vi "UniRec.vi"() -> ()   [LabVIEW 2011]
uses:
  <instrlib>/niHWS/nihws.llb/niHWS Open File Permissions ID.ctl
  <vilib>/DAQmx/write.llb/DAQmx Write (Analog Wfm 1Chan NSamp).vi
  <vilib>/DAQmx/read.llb/DAQmx Read (Analog 1D Wfm NChan NSamp).vi
  <vilib>/DAQmx/create/channels.llb/DAQmx Create Channel (AO-Voltage-Basic).vi
  <vilib>/DAQmx/configure/timing.llb/DAQmx Timing (Sample Clock).vi
  <vilib>/DAQmx/create/channels.llb/DAQmx Create Channel (AI-Voltage-Basic).vi
  <instrlib>/niHWS/nihws.llb/niHWS Write Analog DBL.vi
  <vilib>/DAQmx/miscellaneous.llb/DAQmx Fill In Error Info.vi
  <instrlib>/niHWS/nihws.llb/niHWS Write Analog WDT.vi
  C:/Program Files/National Instruments/LabVIEW 2011/resource/objmgr/daqmx.rc
  <vilib>/gmath/NI_Gmath.lvlib
panel:
  out "File":bool
  in  "low-pass Cut-Off":dbl(knob)=100.0 caption="Lower Cut-Off" scale=2000.0..7000.0 scale format="%#_6p"
  in  "high-pass Cut-Off":dbl(knob)=100.0 caption="Lower Cut-Off" scale=0.0..7000.0 scale format="%#_6p"
  out "data":waveform(dbl)[](array[waveform])
  in  "audio channel":i32
  in  "Audio gain":dbl(knob)=21045.185997761742 scale=0.0..100000.0
  in  "PD gain":dbl=0.001
  out "Waveform Chart 2":waveform(dbl)[](graph)
  in  "Offset":dbl=0.0001
  in  "Record":bool
  in  "Recording Path":path
  in  "Recording channels":tag="4498_1/ai1, 4498_1/ai3, 4498_1/ai5, 4498_1/ai7"
  in  "stop":bool
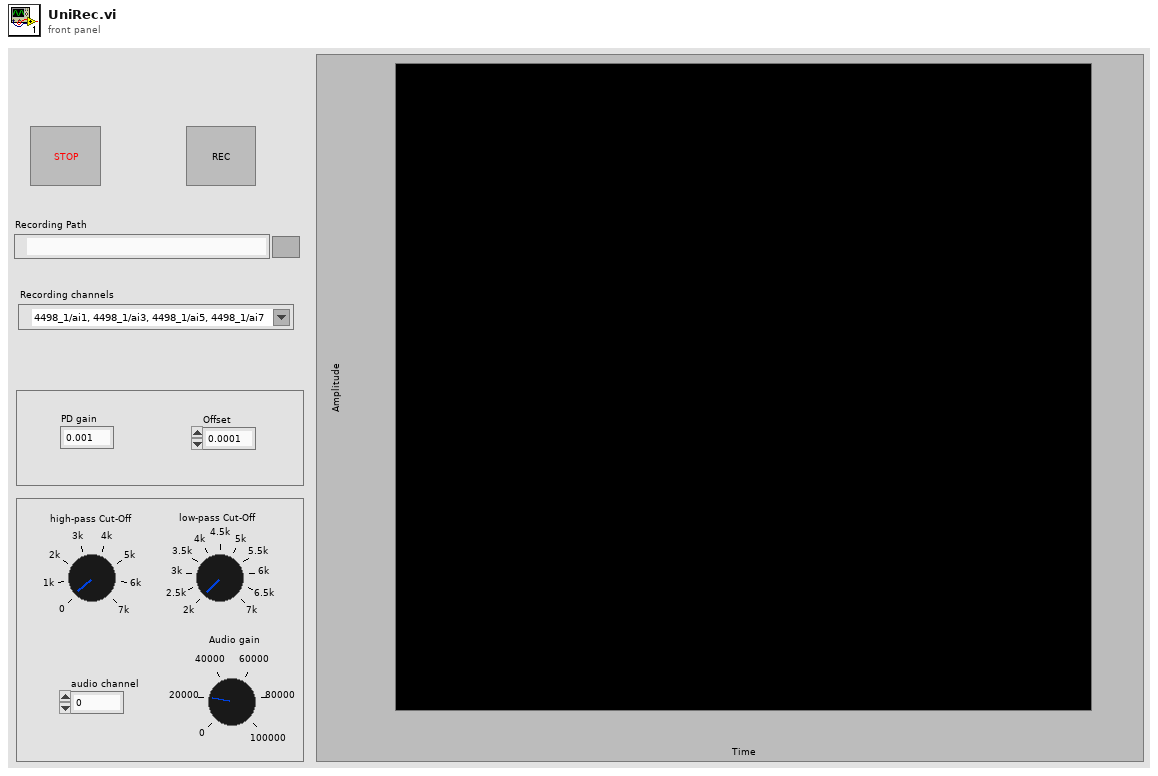
[diagram p1: front panel]
types:
  T1 = typedef "niHWS Open File Permissions ID.ctl" = enum32{"Read Only", "Read/Write Existing", "Read/Write/Create New", "Read/Write/Create New Always"}
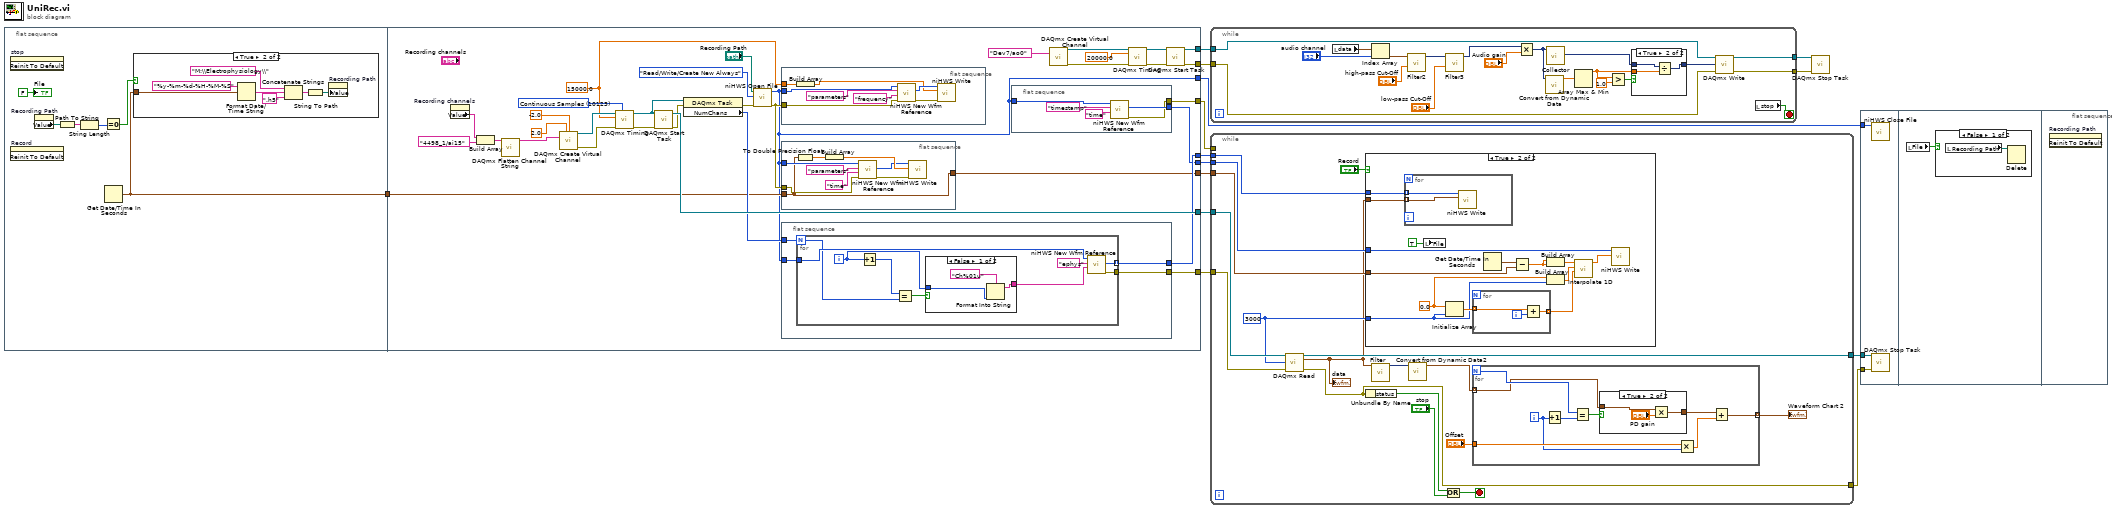
[diagram p0: block diagram]
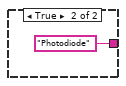
[diagram p5: hidden frame]
diagram:
  n1 = flat-sequence {
    tunnel: [w16] -> w6
    tunnel: [w61] -> w14
    tunnel: [w60] -> w13
    tunnel: [w59] -> w12
    tunnel: [w58] -> w9
    tunnel: [w57] -> w8
    tunnel: [w56] -> w7
    tunnel: w6 -> [w37]
    tunnel: [w30] -> w3
    tunnel: [w29] -> w2
    tunnel: [w28] -> w1
    frame #0 {
      n2 = invoke on="stop" class="Bool (strict)" method="Reinit To Default"() -> ()  [unwired: 3 in, 3 out]
      n3 = invoke on="Record" class="Bool (strict)" method="Reinit To Default"() -> ()  [unwired: 3 in, 3 out]
      n4 = property on="Recording Path" class="Path"() -> ("Value"=w17:path)  [unwired: 2 in, 2 out]
      n5 = Path To String(path=w17) -> (string=w18:string)
      n6 = String Length(string=w18) -> (length=w19:i32)
      n7 = Equal To 0?(x=w19) -> (x = 0?=w20:bool)
      n8 = Get Date/Time In Seconds() -> (seconds since 1Jan1904=w16:timestamp)
      n9 = case shown="True" w20 {
        tunnel: w16 -> [_ w25]
        frame False {
        }
        frame True {
          n10 = Format Date/Time String(time format string (%c)="%y-%m-%d-%H-%M-%S", seconds (now)=w25) -> (date/time string=w22:string)  [unwired: 1 in]
          n11 = Concatenate Strings("M:\\Electrophysiology\\", w22, ".h5") -> (w23:string)
          n12 = String To Path(string=w23) -> (path=w27:path)
          n13 = property on="Recording Path" class="Path"("Value"=w27) -> ()  [unwired: 2 in, 2 out]
        }
      }
      "File" <- FALSE
    }
    frame #1 {
      w52 = 10123 items=["Finite Samples"=10178, "Continuous Samples"=10123, "Hardware Timed Single Point"=12522] ("sample mode")
      w42 = 15000.0 ("rate")
      n14 = property on="Recording channels" class="DAQmxName"() -> ("Value"=w39:string)  [unwired: 2 in, 2 out]
      n15 = Build Array(w39, tag "4498_1/ai15" ("Recording channels 3")) -> (w41:string[])
      n16 = call <vilib>:"DAQmx Flatten Channel String.vi"("names in"=w41) -> ("names out"=w40:string)  [unwired: 13 in, 1 out]
      n17 = call-poly <vilib>:"DAQmx Create Virtual Channel.vi"("maximum value"=2.0, "minimum value"=-2.0, "physical channels"=w40) -> ("task out"=w53:refnum<k21>, "error out"=w51:errorcluster)  [unwired: 11 in]
      n18 = call-poly <vilib>:"DAQmx Timing.vi"("task/channels in"=w53, "sample mode"=w52, "rate"=w42, "error in"=w51) -> ("task out"=w48:refnum<k21>, "error out"=w50:errorcluster)  [unwired: 10 in]
      n19 = call <vilib>:"DAQmx Start Task.vi"("task/channels in"=w48, "error in"=w50) -> ("task out"=w61:refnum<k21>, "error out"=w49:errorcluster)  [unwired: 12 in]
      n20 = property class="DAQmx Task"(reference=w48, error in=w49) -> (error out=w45:errorcluster, "NumChans"=w43:u32)  [unwired: 1 out]
      n21 = call <instrlib>:"niHWS Open File.vi"("error in (no error)"=w45, "permissions (0:read only)"=niHWS_Open_File_Permissions_ID."Read/Write/Create New Always", "file path"="Recording Path") -> ("error out"=w44:errorcluster, "file handle"=w28:u32)  [unwired: 7 in]
      n22 = flat-sequence {
        tunnel: w42 -> [w79]
        tunnel: w44 -> [w78]
        tunnel: w28 -> [w77]
        frame #0 {
          n23 = Build Array(w79) -> (w80:dbl[])
          n24 = call <instrlib>:"niHWS New Wfm Reference.vi"("error in (no error)"=w78, "waveform name (empty)"="frequency" ("group name (empty)"), "group name (empty)"="parameters", "file handle in"=w77) -> ("error out"=w76:errorcluster, "waveform reference"=w83:u32)  [unwired: 5 in, 1 out]
          n25 = call-poly <instrlib>:"niHWS Write.vi"("error in (no error)"=w76, "data"=w80, "waveform reference in"=w83) -> ()  [unwired: 7 in, 2 out]
        }
      }
      n26 = flat-sequence {
        tunnel: w44 -> [w75]
        tunnel: w28 -> [w74]
        tunnel: [w67] -> w56
        tunnel: w37 -> [w67]
        frame #0 {
          n27 = To Double Precision Float(number=w67) -> (double precision float=w73:dbl)
          n28 = Build Array(w73) -> (w72:dbl[])
          n29 = call <instrlib>:"niHWS New Wfm Reference.vi"("error in (no error)"=w75, "waveform name (empty)"="time" ("group name (empty)"), "group name (empty)"="parameters", "file handle in"=w74) -> ("error out"=w68:errorcluster, "waveform reference"=w69:u32)  [unwired: 5 in, 1 out]
          n30 = call-poly <instrlib>:"niHWS Write.vi"("error in (no error)"=w68, "data"=w72, "waveform reference in"=w69) -> ()  [unwired: 7 in, 2 out]
        }
      }
      n31 = flat-sequence {
        tunnel: w43 -> [w86]
        tunnel: w28 -> [w87]
        tunnel: [w85] -> w60
        tunnel: [w84] -> w59
        frame #0 {
          n32 = for {
            N: w86 -> [w91]
            tunnel: [w93] -> w85 mode=indexing
            tunnel: [w92] -> w84
            tunnel: w87 -> [w96]
            i -> [w90]
            n33 = Increment(x=w90) -> (x+1=w89:i32)
            n34 = Equal?(x=w89, y=w91) -> (x = y?=w88:bool)
            n35 = case shown="False" w88 {
              tunnel: w90 -> [w99 _]
              tunnel: [w97 "Photodiode"] -> w94
              frame False {
                n36 = Format Into String(format string="Ch%01u", w99) -> (resulting string=w97:string)  [unwired: 2 in, 1 out]
              }
              frame True {
              }
            }
            n37 = call <instrlib>:"niHWS New Wfm Reference.vi"("waveform name (empty)"=w94, "group name (empty)"="ephys", "file handle in"=w96) -> ("error out"=w92:errorcluster, "waveform reference"=w93:u32)  [unwired: 6 in, 1 out]
          }
        }
      }
      n38 = flat-sequence {
        tunnel: [w66] -> w58
        tunnel: [w65] -> w57
        tunnel: w28 -> [w63]
        frame #0 {
          n39 = call <instrlib>:"niHWS New Wfm Reference.vi"("waveform name (empty)"="time" ("format string"), "group name (empty)"="timestamp", "file handle in"=w63) -> ("error out"=w65:errorcluster, "waveform reference"=w66:u32)  [unwired: 6 in, 1 out]
        }
      }
      n40 = call-poly <vilib>:"DAQmx Create Virtual Channel.vi"("physical channels"=tag "Dev7/ao0") -> ("task out"=w35:refnum<k21>, "error out"=w32:errorcluster)  [unwired: 13 in]
      n41 = call-poly <vilib>:"DAQmx Timing.vi"("task/channels in"=w35, "rate"=20000.0, "error in"=w32) -> ("task out"=w33:refnum<k21>, "error out"=w31:errorcluster)  [unwired: 11 in]
      n42 = call <vilib>:"DAQmx Start Task.vi"("task/channels in"=w33, "error in"=w31) -> ("task out"=w30:refnum<k21>, "error out"=w29:errorcluster)  [unwired: 12 in]
    }
  }
  n43 = while {
    tunnel: [w115] -> w5
    tunnel: [w114] -> w4
    tunnel: w3 -> [w113]
    tunnel: w2 -> [w112]
    stop <- w116 stop-if-true
    n44 = local read "data"() -> (w109:waveform(dbl)[])
    n45 = Index Array(array=w109, index="audio channel") -> (element=w104:waveform(dbl))
    n46 = call "Filter2"("Lower Cut-Off"="high-pass Cut-Off", "Signal"=w104) -> ("Filtered Signal"=w105:dynamicdata)  [unwired: 8 in, 1 out]
    n47 = call "Filter3"("Lower Cut-Off"="low-pass Cut-Off", "Signal"=w105) -> ("Filtered Signal"=w103:dynamicdata)  [unwired: 8 in, 1 out]
    n48 = Multiply(x=w103, y="Audio gain") -> (x*y=w102:dynamicdata)
    n49 = call "Convert from Dynamic Data"("Dynamic Data Type"=w102) -> ("Array"=w120:dbl[])  [unwired: 3 in]
    n50 = call "Collector"("Signals"=w102) -> ("Collected Signals"=w101:dynamicdata)  [unwired: 9 in, 1 out]
    n51 = Array Max & Min(array=w120) -> (max value=w117:dbl)  [unwired: 3 out]
    n52 = Greater?(x=w117, y=1.0) -> (0:w118:bool)
    n53 = case shown="True" w118 {
      tunnel: w101 -> [w121 w124]
      tunnel: [w121 w122] -> w110
      tunnel: w117 -> [_ w123]
      frame False {
      }
      frame True {
        n54 = Divide(x=w124, y=w123) -> (x/y=w122:dynamicdata)
      }
    }
    n55 = call-poly <vilib>:"DAQmx Write.vi"("task/channels in"=w113, "data"=w110, "error in"=w112) -> ("task out"=w115:refnum<k21>, "error out"=w114:errorcluster)  [unwired: 10 in, 1 out]
    n56 = local read "stop"() -> (w116:bool)
  }
  n57 = while {
    tunnel: w14 -> [w139]
    tunnel: w13 -> [w134]
    tunnel: w12 -> [w138]
    tunnel: [w137] -> w11
    tunnel: [w129] -> w10
    tunnel: w9 -> [w133]
    tunnel: w8 -> [_]
    tunnel: w7 -> [w132]
    stop <- w141 stop-if-true
    w130 = 3000 ("number of samples per channel")
    n58 = call-poly <vilib>:"DAQmx Read.vi"("task/channels in"=w139, "number of samples per channel"=w130, "error in"=w138) -> ("task out"=w137:refnum<k21>, "data"=w127:waveform(dbl)[], "error out"=w129:errorcluster)  [unwired: 10 in]
    "data" <- w127
    n59 = case shown="True" "Record" {
      tunnel: w127 -> [_ w165]
      tunnel: w134 -> [_ w168]
      tunnel: w133 -> [_ w156]
      tunnel: w132 -> [_ w166]
      tunnel: w130 -> [_ w159]
      frame False {
      }
      frame True {
        w158 = 0.0 ("element")
        n60 = for {
          tunnel: w165 -> [w173] mode=indexing
          tunnel: w168 -> [w172] mode=indexing
          n61 = call-poly <instrlib>:"niHWS Write.vi"("analog waveform"=w173, "waveform reference in"=w172) -> ()  [unwired: 8 in, 2 out]
        }
        n62 = local write "File"(TRUE) -> ()
        n63 = Initialize Array(w158, w159) -> (w160:dbl[])
        n64 = for {
          tunnel: w160 -> [w171] mode=indexing
          tunnel: [w169] -> w157 mode=indexing
          i -> [w170]
          n65 = Add(x=w171, y=w170) -> (x+y=w169:dbl)
        }
        n66 = Get Date/Time In Seconds() -> (seconds since 1Jan1904=w167:timestamp)
        n67 = Subtract(x=w167, y=w166) -> (x-y=w164:dbl)
        n68 = Build Array(w164, w164) -> (w163:dbl[])
        n69 = Build Array(w158, w159) -> (w161:dbl[])
        n70 = call <vilib>:"Interpolate 1D.vi"("xi"=w157, "X"=w161, "Y"=w163) -> ("yi"=w162:dbl[])  [unwired: 6 in, 2 out]
        n71 = call-poly <instrlib>:"niHWS Write.vi"("data"=w162, "waveform reference in"=w156) -> ()  [unwired: 8 in, 2 out]
      }
    }
    n72 = Unbundle By Name(w129) -> ("status"=w136:bool)
    n73 = call "Filter"("Signal"=w127) -> ("Filtered Signal"=w126:dynamicdata)  [unwired: 9 in, 1 out]
    n74 = call "Convert from Dynamic Data2"("Dynamic Data Type"=w126) -> ("Array of Waveform"=w125:waveform(dbl)[])  [unwired: 3 in]
    n75 = Or(x=w136, y="stop") -> (x .or. y?=w141:bool)
    n76 = for {
      N -> [w148]
      tunnel: "Offset" -> [w150]
      tunnel: [w142] -> w128 mode=indexing
      tunnel: w125 -> [w143] mode=indexing
      i -> [w144]
      n77 = Increment(x=w144) -> (x+1=w147:i32)
      n78 = Equal?(x=w148, y=w147) -> (x = y?=w146:bool)
      n79 = case shown="True" w146 {
        tunnel: w143 -> [w151 w153]
        tunnel: [w151 w152] -> w145
        frame False {
        }
        frame True {
          n80 = Multiply(x=w153, y="PD gain") -> (x*y=w152:waveform(dbl))
        }
      }
      n81 = Multiply(x=w150, y=w144) -> (x*y=w149:dbl)
      n82 = Add(x=w145, y=w149) -> (x+y=w142:waveform(dbl))
    }
    "Waveform Chart 2" <- w128
  }
  n83 = call <vilib>:"DAQmx Stop Task.vi"("task/channels in"=w5, "error in"=w4) -> ()  [unwired: 12 in, 2 out]
  n84 = flat-sequence {
    tunnel: w11 -> [w176]
    tunnel: w10 -> [w175]
    tunnel: w1 -> [w174]
    frame #0 {
      n85 = call <instrlib>:"niHWS Close File.vi"("file handle"=w174) -> ()  [unwired: 10 in, 1 out]
      n86 = call <vilib>:"DAQmx Stop Task.vi"("task/channels in"=w176, "error in"=w175) -> ()  [unwired: 12 in, 2 out]
    }
    frame #1 {
      n87 = local read "File"() -> (w177:bool)
      n88 = case shown="False" w177 {
        frame False {
          n89 = local read "Recording Path"() -> (w178:path)
          n90 = Delete(path (use dialog)=w178) -> ()  [unwired: 4 in, 3 out]
        }
        frame True {
        }
      }
    }
    frame #2 {
      n91 = invoke on="Recording Path" class="Path" method="Reinit To Default"() -> ()  [unwired: 3 in, 3 out]
    }
  }
